vi "niDTS GNSS RF Test Full Example.vi"() -> ()   [LabVIEW 2014]
uses:
  GPS Rx RF Test/Includes/niDTS GNSS GPS Rx RF Test INC Results.ctl
  GPS Rx RF Test/Includes/niDTS GNSS GPS Rx RF Test INC Parameters.ctl
  GPS Rx RF Test/Includes/niDTS GNSS GPS Rx RF Test INC Channel.ctl
  TestStand/Station/Objects/SystemDutHandle/Includes/niDTS SystemDutHandle INC SystemDutHandles.ctl
  TestStand/Station/Objects/SystemDutHandle/niDTS SystemDutHandle.lvclass
  Framework/Dut/Includes/niDTS Dut INC Handle.ctl
  Framework/Dut/Objects/BASE_class/niDTS Dut.lvclass
  TestStand/Station/Objects/SystemTechnologyCatalog/niDTS SystemTechnologyCatalog.lvclass
  TestStand/Station/Objects/SystemDut/niDTS SystemDut.lvclass
  Framework/niDTS Framework.lvlib
  TestStand/niDTS TestStand.lvlib
  Plugins/niWTM Loopback/niWTM Loopback.lvlib
  Framework/Logger/Listener/Viewer/niDTS Logger Listener Viewer.lvclass
  niDTS GNSS.lvlib
panel:
  in  "Results":enum32{"GPS"}(tab)
  out "GPS Results":T1
  in  "Keep Log Open":bool
  in  "ResultsIndex":u8=1
  in  "System Configuration XML Path":path=path "C:/Users/Public/Documents/National Instruments/WTM 1.0/System Configurations"
  in  "Socket Index":i32
  out "error out":errorcluster
  in  "DUT Config":enum32{"Loopback"}(tab)
  in  "Socket Parameters":T2={"GNSS"={"VISA Resource"="TCPIP0::InstrumentAddress::inst0::INSTR", "PortNames "=["Port0"]}}
  in  "Test Config":enum32{"GPS"}(tab)
  in  "GPS":T3={"Channel"=enum."L1 - 1575.42 MHz", "Power (dBm)"=0.0, "External Attenuation (dB)"=0.0, "Measurement Interval (s)"=0.005, "Number of Averages"=1, "Waveform Name"="GPS_100Bits_1Sat.tdms"} {"External Attenuation (dB)" format="%.1g"; "Power (dBm)" format="%.1g"}
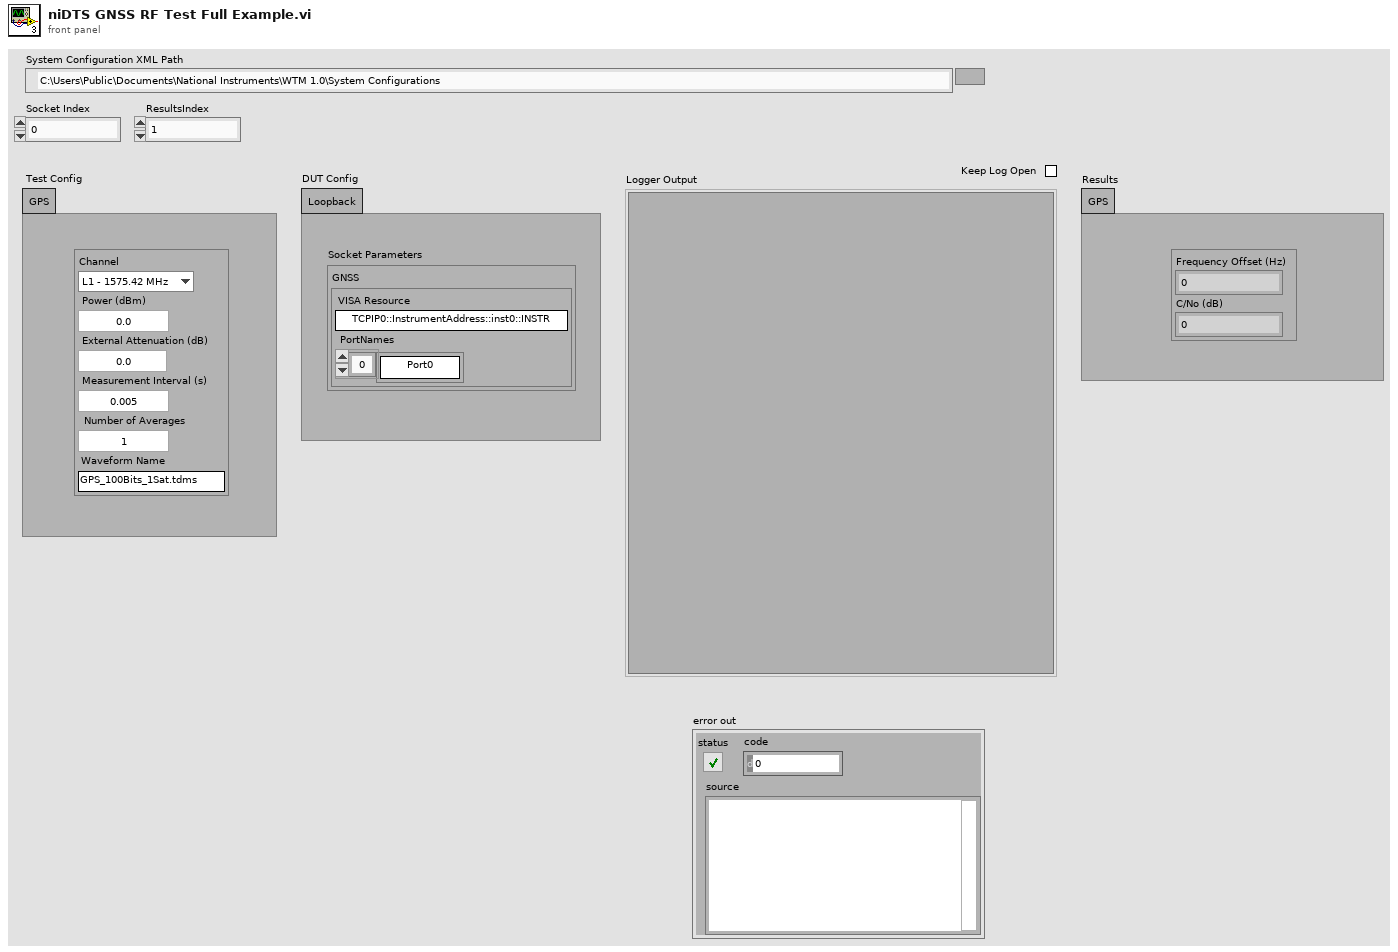
[diagram p1: front panel]
types:
  T1 = typedef "niDTS GNSS.lvlib/niDTS GNSS GPS Rx RF Test INC Results.ctl" = cluster{"Frequency Offset (Hz)":dbl, "C/No (dB)":dbl}
  T2 = cluster{"GNSS":cluster{"VISA Resource":string, "PortNames ":string[]}}
  T3 = typedef "niDTS GNSS.lvlib/niDTS GNSS GPS Rx RF Test INC Parameters.ctl" = cluster{"Channel":T4, "Power (dBm)":dbl, "External Attenuation (dB)":dbl, "Measurement Interval (s)":dbl, "Number of Averages":i32, "Waveform Name":string}
  T4 = typedef "niDTS GNSS.lvlib/niDTS GNSS GPS Rx RF Test INC Channel.ctl" = enum16{"L1 - 1575.42 MHz", "L2 - 1227.60 MHz", "L5 - 1176.45 MHz"}
  T5 = cluster{"WLAN":cluster{"VISA Resource":string, "PortNames ":string[]}, "Bluetooth":cluster{"VISA Resource":string, "PortNames ":string[]}, "GNSS":cluster{"VISA Resource":string, "PortNames ":string[]}}
  T6 = cluster{"WLAN":cluster{"idle interval":dbl, "Payload Length Limit":i32, "Channel Secondary Factor":enum16{"-1", "1", "0"}}}
  T7 = typedef "niDTS Framework.lvlib/niDTS Dut INC Handle.ctl" = refnum<data-value>
  T8 = typedef "niDTS TestStand.lvlib/niDTS SystemDutHandle.lvclass/niDTS SystemDutHandle INC SystemDutHandles.ctl" = refnum<class "niDTS SystemDutHandle.lvclass">[]
  T9 = typedef "niDTS Framework.lvlib/niDTS Logger INC Handle.ctl" = refnum<data-value>
  T10 = cluster{"VISA Resource":string, "PortNames ":string[]}
  T11 = typedef "niDTS GNSS.lvlib/niDTS GNSS RF Test INC Handle.ctl" = refnum<data-value>
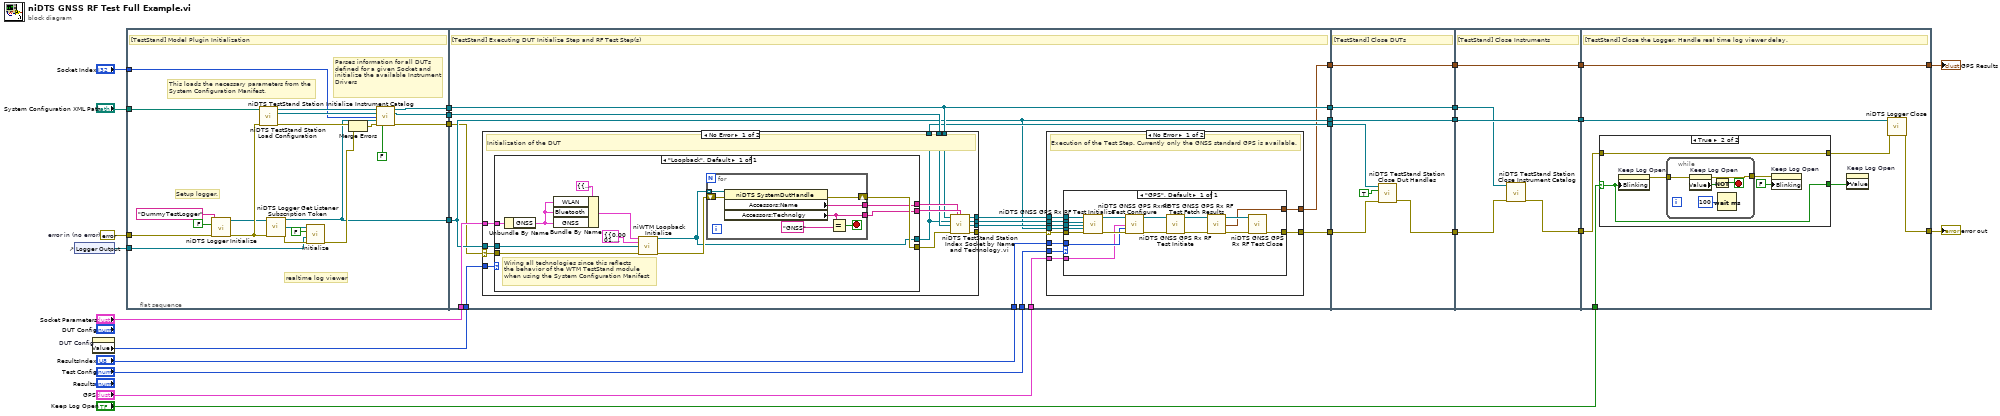
[diagram p0: block diagram]
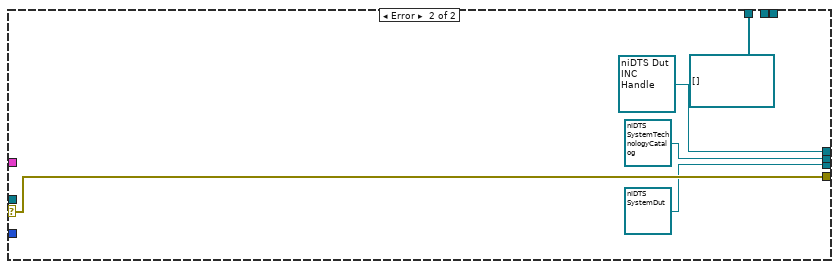
[diagram p2: hidden frame]
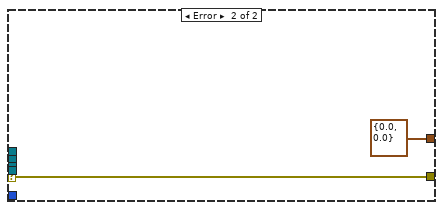
[diagram p3: hidden frame]
diagram:
  w22 = errorcluster {"status"=FALSE, "code"=0, "source"=""}  # error in (no error)
  n1 = control-ref of="Logger Output"() -> (w21:refnum<vi>)
  n2 = property on="DUT Config" class="TabCtl (strict)"() -> ("Value"=w7:enum32{"Loopback"})  [unwired: 2 in, 2 out]
  n3 = flat-sequence {
    tunnel: [w36] -> w28
    tunnel: [w35] -> w27
    tunnel: [w34] -> w26
    tunnel: [w33] -> w25
    tunnel: "Socket Index" -> [w32]
    tunnel: "System Configuration XML Path" -> [w31]
    tunnel: w22 -> [w30]
    tunnel: w21 -> [w29]
    tunnel: w28 -> [w61]
    tunnel: w27 -> [w62]
    tunnel: w26 -> [w51]
    tunnel: w25 -> [w56]
    tunnel: "Socket Parameters" -> [w60]
    tunnel: w7 -> [w59]
    tunnel: [w61] -> w20
    tunnel: [w58] -> w18
    tunnel: [w57] -> w16
    tunnel: [w56] -> w15
    tunnel: "ResultsIndex" -> [w53]
    tunnel: "Test Config" -> [w55]
    tunnel: "GPS" -> [w54]
    tunnel: [w50] -> w3
    tunnel: w20 -> [w139]
    tunnel: [w139] -> w19
    tunnel: w18 -> [w135]
    tunnel: [w134] -> w17
    tunnel: w16 -> [w136]
    tunnel: w15 -> [w138]
    tunnel: [w138] -> w14
    tunnel: [w133] -> w4
    tunnel: w3 -> [w133]
    tunnel: w19 -> [w142]
    tunnel: w17 -> [w141]
    tunnel: w14 -> [w144]
    tunnel: [w144] -> w13
    tunnel: [w143] -> w12
    tunnel: [w140] -> w5
    tunnel: w4 -> [w140]
    tunnel: [w148] -> w11
    tunnel: w13 -> [w151]
    tunnel: w12 -> [w149]
    tunnel: "Keep Log Open" -> [w147]
    tunnel: w5 -> [w146]
    tunnel: [w146] -> w2
    frame #0 {
      # "Setup logger."
      # "realtime log viewer"
      # "Parses information for all DUTs defined for a given Socket and \ninitialize the available Instrument\nDrivers"
      # "This loads the necessary parameters from the \nSystem Configuration Manifest."
      # "[TestStand] Model Plugin Initialization"
      n4 = call "niDTS Logger Initialize.vi"("Session Name ()"="DummyTestLogger", "Log to File"=FALSE, "error in (no error)"=w30) -> ("Logger Handle out"=w45:T9, "error out"=w46:errorcluster)  [unwired: 11 in]
      n5 = call "niDTS TestStand Station Load Configuration.vi"("System Configuration XML Path"=w31, "error in (no error)"=w46) -> ("All System Hardware"=w41:refnum<class "niDTS SystemHardware.lvclass">, "All DUT Definitions"=w39:refnum<class "niDTS SystemDut.lvclass">[], "error out"=w48:errorcluster)  [unwired: 11 in]
      n6 = call "niDTS Logger Get Listener Subscription Token.vi"("Logger Handle in"=w45, "error in (no error)"=w46) -> ("Logger Handle out"=w33:T9, "Listener Subscription Token"=w42:refnum<class "niDTS Logger Listener Subscription Token.lvclass">, "error out"=w43:errorcluster)  [unwired: 11 in]
      n7 = call "Initialize.vi"("error in (no error)"=w43, "SubPanel Reference"=w29, "Open Viewer?"=FALSE, "Listener Subscription Token"=w42) -> ("error out"=w49:errorcluster)  [unwired: 6 in, 1 out]
      n8 = Merge Errors(w48, w49) -> (w47:errorcluster)
      n9 = call "niDTS TestStand Station Initialize Instrument Catalog.vi"("All System Hardware"=w41, "All DUT Definitions"=w39, "Socket Index"=w32, "Logger Handle"=w33, "error in (no error)"=w47, "Simulation Mode (F)"=FALSE) -> ("Socket Instrument Catalog"=w36:refnum<class "niDTS SystemInstrCatalog.lvclass">, "Socket DUT Definitions"=w35:refnum<class "niDTS SystemDut.lvclass">[], "error out"=w34:errorcluster)  [unwired: 7 in]
    }
    frame #1 {
      # "[TestStand] Executing DUT Initialize Step and RF Test Step(s)"
      n10 = case shown="No Error" w51 {
        selector: w51 -> [w66 w103]
        tunnel: [w77 refnum<class "niDTS SystemDut.lvclass"> refnum ("Specific Socket/Tech DUT Definition")] -> w65
        tunnel: [w76 refnum<class "niDTS SystemTechnologyCatalog.lvclass"> refnum ("SystemTechnologyCatalog")] -> w64
        tunnel: [w75 T7 refnum ("Dut Handle")] -> w63
        tunnel: w62 -> [w74 _]
        tunnel: w61 -> [w73 _]
        tunnel: w60 -> [w72 _]
        tunnel: w59 -> [w71 _]
        tunnel: [w70 T8 [] ("Dut Technology Handles")] -> w57
        tunnel: w56 -> [w69 _]
        tunnel: [w68 w103] -> w52
        frame No Error {
          # "Initialization of the DUT"
          n11 = case shown="\"Loopback\", Default" w71 {
            tunnel: [w83] -> w67
            tunnel: w69 -> [w90]
            tunnel: [w80] -> w70
            tunnel: [w82] -> w78
            tunnel: [w81] -> w79
            tunnel: w72 -> [w88]
            tunnel: w66 -> [w89]
            frame "Loopback", Default {
              # "Wiring all technologies since this reflects \nthe behavior of the WTM TestStand module \nwhen using the System Configuration Manifest"
              n12 = Unbundle By Name(w88) -> ("GNSS"=w86:T10)
              n13 = Bundle By Name(cluster=T5 {"WLAN"={"VISA Resource"="TCPIP0::InstrumentAddress::inst0::INSTR", "PortNames "=["Port0"]}, "Bluetooth"={"VISA Resource"="TCPIP0::InstrumentAddress::inst0::INSTR", "PortNames "=["Port0"]}, "GNSS"={"VISA Resource"="TCPIP0::InstrumentAddress::inst0::INSTR", "PortNames "=["Port0"]}} ("Socket Parameters"), "WLAN"=w86, "Bluetooth"=w86, "GNSS"=w86) -> (w85:T5)
              n14 = call "niWTM Loopback Initialize.vi"("Socket Parameters"=w85, "General Parameters"=T6 {"WLAN"={"idle interval"=0.0001, "Payload Length Limit"=12000, "Channel Secondary Factor"=enum."0"}} ("General Parameters niWTM Loopback"), "Logger"=w90, "error in (no error)"=w89) -> ("Dut Technology Handles"=w80:T8, "error out"=w84:errorcluster)  [unwired: 10 in]
              n15 = for {
                tunnel: [w93] -> w81
                tunnel: [w96] -> w82
                shift-right: [w97] -> w83
                shift-left: w84 -> [w98]
                tunnel: w80 -> [w95] mode=indexing
                stop <- w92 stop-if-true
                n16 = property class="niDTS SystemDutHandle"(reference=w95, error in=w98) -> (error out=w97:errorcluster, "Accessors:Name"=w96:string, "Accessors:Technolgy"=w93:string)  [unwired: 1 out]
                n17 = Equal?(x=w93, y="GNSS") -> (x = y?=w92:bool)
              }
            }
          }
          n18 = call "niDTS TestStand Station Index Socket by Name and Technology,vi.vi"("niDTS SystemInstrCatalog in"=w73, "Name"=w78, "Technology"=w79, "System Dut Handles"=w70, "Socket DUT Definitions"=w74, "error in (no error)"=w67) -> ("Dut Handle"=w75:T7, "SystemTechnologyCatalog"=w76:refnum<class "niDTS SystemTechnologyCatalog.lvclass">, "Specific Socket/Tech DUT Definition"=w77:refnum<class "niDTS SystemDut.lvclass">, "error out"=w68:errorcluster)  [unwired: 6 in]
        }
        frame Error {
        }
      }
      n19 = case shown="No Error" w52 {
        selector: w52 -> [w105 w132]
        tunnel: w65 -> [w113 _]
        tunnel: w64 -> [w112 _]
        tunnel: w63 -> [w111 _]
        tunnel: [w110 w132] -> w58
        tunnel: w56 -> [w109 _]
        tunnel: w55 -> [w108 _]
        tunnel: w54 -> [w107 _]
        tunnel: w53 -> [w106 _]
        tunnel: [w104 T1 {"Frequency Offset (Hz)"=0.0, "C/No (dB)"=0.0} ("GPS Results")] -> w50
        frame No Error {
          # "Execution of the Test Step. Currently only the GNSS standard GPS is available."
          n20 = case shown="\"GPS\", Default" w108 {
            tunnel: [w122] -> w110
            tunnel: w105 -> [w123]
            tunnel: w109 -> [w121]
            tunnel: w111 -> [w120]
            tunnel: w112 -> [w119]
            tunnel: w113 -> [w118]
            tunnel: w106 -> [w117]
            tunnel: [w115] -> w104
            tunnel: w107 -> [w114]
            frame "GPS", Default {
              n21 = call "niDTS GNSS GPS Rx RF Test Initialize.vi"("Dut Reference"=w120, "SystemTechnologyCatalog"=w119, "SystemDut"=w118, "Logger Reference"=w121, "error in (no error)"=w123) -> ("Dummy Test Handle out"=w124:T11, "error out"=w125:errorcluster)  [unwired: 8 in, 1 out]
              n22 = call "niDTS GNSS GPS Rx RF Test Configure.vi"("Template Tx Test Handle in"=w124, "Parameters"=w114, "ResultsIndex"=w117, "error in (no error)"=w125) -> ("Template Tx Test Handle out"=w127:T11, "error out"=w128:errorcluster)  [unwired: 10 in]
              n23 = call "niDTS GNSS GPS Rx RF Test Initiate.vi"("Template Tx Test Handle in"=w127, "error in (no error)"=w128) -> ("Template Tx Test Handle out"=w130:T11, "error out"=w126:errorcluster)  [unwired: 12 in]
              n24 = call "niDTS GNSS GPS Rx RF Test Fetch Results.vi"("Template Tx Test Handle in"=w130, "error in (no error)"=w126) -> ("Template Tx Test Handle out"=w116:T11, "GPS Results"=w115:T1, "error out"=w129:errorcluster)  [unwired: 11 in]
              n25 = call "niDTS GNSS GPS Rx RF Test Close.vi"("Template Tx Test Handle"=w116, "error in (no error)"=w129) -> ("error out"=w122:errorcluster)  [unwired: 13 in]
            }
          }
        }
        frame Error {
        }
      }
    }
    frame #2 {
      # "[TestStand] Close DUTs"
      n26 = call "niDTS TestStand Station Close Dut Handles.vi"("Socket Dut Handles In"=w136, "Close All"=TRUE, "error in (no error)"=w135) -> ("error out"=w134:errorcluster)  [unwired: 11 in, 1 out]
    }
    frame #3 {
      # "[TestStand] Close Instruments"
      n27 = call "niDTS TestStand Station Close Instrument Catalog.vi"("Socket Instrument Catalog"=w142, "error in (no error)"=w141) -> ("error out"=w143:errorcluster)  [unwired: 13 in]
    }
    frame #4 {
      # "[TestStand] Close the Logger. Handle real time log viewer delay."
      n28 = case shown="True" w147 {
        selector: w147 -> [w152 w154]
        tunnel: w149 -> [w153 w158]
        tunnel: [w153 w158] -> w150
        tunnel: [w152 w154] -> w145
        frame False {
        }
        frame True {
          n29 = property on="Keep Log Open" class="Bool (strict)"("Blinking"=w154) -> (error out=w155:errorcluster)  [unwired: 2 in, 1 out]
          n30 = while {
            tunnel: [w162] -> w156
            tunnel: w155 -> [w161]
            stop <- w160 stop-if-true
            n31 = property on="Keep Log Open" class="Bool (strict)"(error in=w161) -> (error out=w162:errorcluster, "Value"=w159:bool)  [unwired: 1 in, 1 out]
            n32 = Not(x=w159) -> (.not. x?=w160:bool)
            n33 = Wait (ms)(milliseconds to wait=u32 100) -> ()  [unwired: 1 out]
          }
          n34 = property on="Keep Log Open" class="Bool (strict)"(error in=w156, "Blinking"=FALSE) -> ()  [unwired: 1 in, 2 out]
        }
      }
      n35 = property on="Keep Log Open" class="Bool (strict)"("Value"=w145) -> ()  [unwired: 2 in, 2 out]
      n36 = call "niDTS Logger Close.vi"("Logger Handle in"=w151, "error in (no error)"=w150) -> ("error out"=w148:errorcluster)  [unwired: 13 in]
    }
  }
  "error out" <- w11
  "GPS Results" <- w2
